vi "fill-append.vi"(2 "Append/Fill":bool caption="Append=Tl", 3 "array":dbl[](array[numeric]), 4 "Steps (max 200)":i32=200 max=200, 5 "To":dbl=1.2, 6 "From":dbl=-1.2) -> (0 "appended magnetic field values":dbl[](array[numeric]))   [LabVIEW 2023]
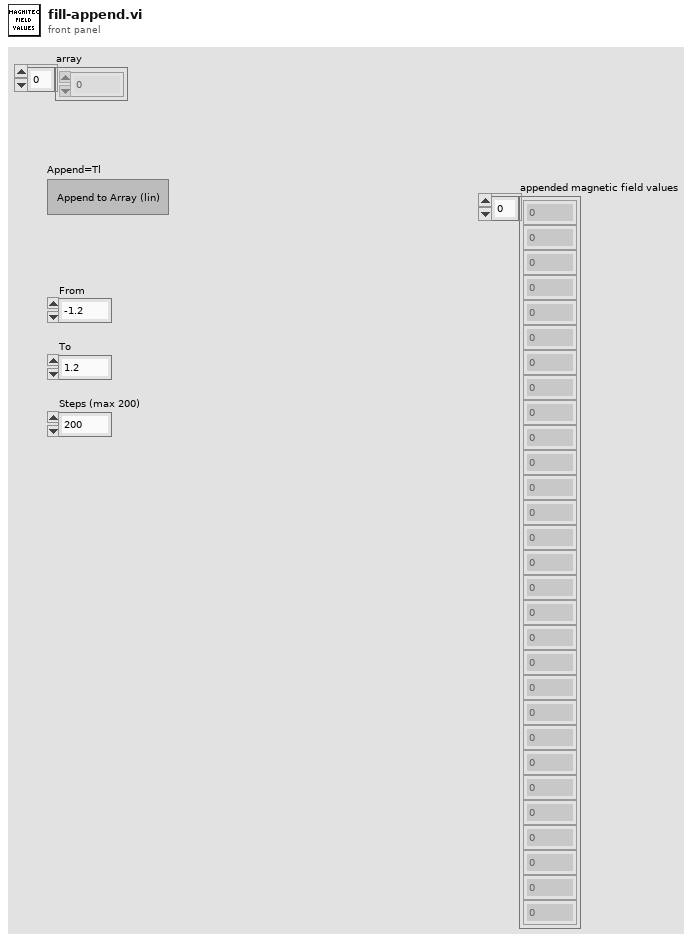
[diagram p1: front panel]
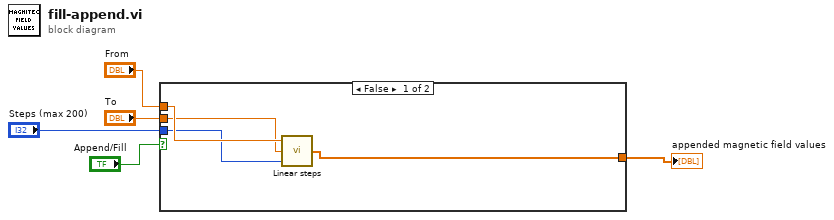
[diagram p0: block diagram]
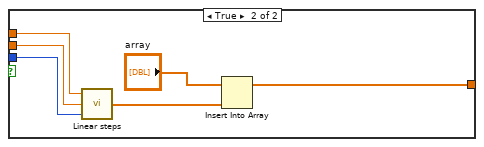
[diagram p2: hidden frame]
diagram:
  n1 = case shown="False" "Append/Fill" {
    tunnel: "From" -> [w9 w15]
    tunnel: "To" -> [w8 w14]
    tunnel: "Steps (max 200)" -> [w7 w13]
    tunnel: [w6 w11] -> w5
    frame False {
      n2 = call "Linear steps.vi"("Steps"=w7, "To"=w8, "From"=w9) -> ("Array"=w6:dbl[])
    }
    frame True {
      n3 = call "Linear steps.vi"("Steps"=w13, "To"=w14, "From"=w15) -> ("Array"=w12:dbl[])
      n4 = Insert Into Array(array="array", new element=w12) -> (w11:dbl[])  [unwired: 1 in]
    }
  }
  "appended magnetic field values" <- w5
